vi "GenNet Check Connection.vi"(4 "local port (0)":u16, 6 "timeout [ms]":i32=100, 8 "error in (no error)":errorcluster, 9 "remote port":u16, 10 "ip address":string, 11 "TCP Network Connection in":refnum<k5>) -> (0 "error out":errorcluster, 3 "TCP Network Connection out":refnum<k5>)   [LabVIEW 2014, in "hse-gennet.lvlib"]
doc: "Checks for a valid TCP/IP connection. Reestablishes the connection if no valid connection found. Creates a new connection if none was given.\n\n____\nHAMPEL SOFTWARE ENGINEERING v0.7.0 (2018-07-16 18:12)"
uses:
  hse-gennet.lvlib
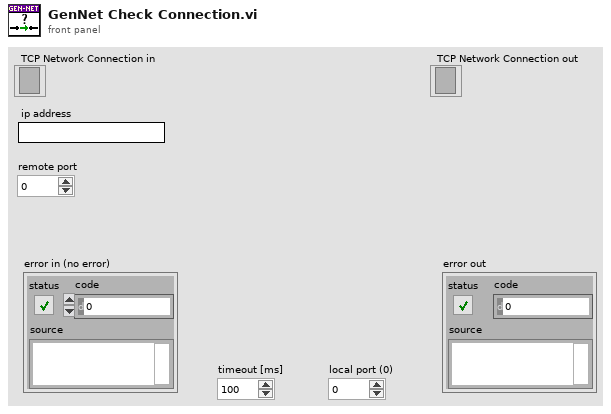
[diagram p1: front panel]
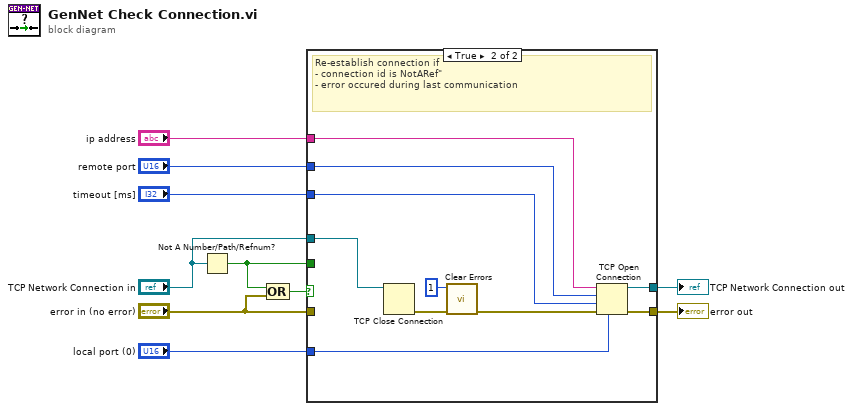
[diagram p0: block diagram]
diagram:
  n1 = Not A Number/Path/Refnum?(number/path/refnum="TCP Network Connection in") -> (NaN/Path/Refnum?=w2:bool)
  n2 = Compound Arithmetic op=OR(w2, "error in (no error)") -> (w4:bool)
  n3 = case shown="True" w4 {
    tunnel: [w11 w22] -> w10
    tunnel: [w12 w20] -> w9
    tunnel: "error in (no error)" -> [w12 _]
    tunnel: "local port (0)" -> [_ w19]
    tunnel: "timeout [ms]" -> [_ w18]
    tunnel: "remote port" -> [_ w17]
    tunnel: "ip address" -> [_ w16]
    tunnel: "TCP Network Connection in" -> [w11 w13]
    tunnel: w2 -> [_ _]
    frame False {
      # "Use existing connection"
    }
    frame True {
      # "Re-establish connection if \n- connection id is NotARef\"\n- error occured during last communication"
      n4 = TCP Close Connection(connection ID=w13) -> (error out=w21:errorcluster)  [unwired: 1 in, 2 out]
      n5 = call <vilib>:"Clear Errors.vi"("error in (no error)"=w21, "specific error code to clear (0: all)"=1) -> ("error out"=w15:errorcluster)  [unwired: 4 in, 1 out]
      n6 = TCP Open Connection(address=w16, remote port or service name=w17, timeout ms (60000)=w18, local port=w19, error in (no error)=w15) -> (connection ID=w22:refnum<k5>, error out=w20:errorcluster)
    }
  }
  "TCP Network Connection out" <- w10
  "error out" <- w9
